vi "Actor Core.vi"(8 "error in":errorcluster, 11 "RandomDataChart in":refnum<class "ButtonPanel.lvclass">) -> (0 "error out":errorcluster, 3 "Actor out":refnum<class "Actor.lvclass">)   [LabVIEW 2015, in "TestActors.lvlib" / "ButtonPanel.lvclass"]
doc: "(<B>Filename</B>: Actor Framework.lvlib:Actor.lvclass:Actor Core.vi)\n\nReceives messages to the actor, reacts to them, and initiates any error handling that may shut the actor down.\n\nDescendant classes may override this VI to append parallel tasks for the actor to complete while it handles messages. Overrides use the Call Parent Method node."
uses:
  ButtonPanel.lvclass
  <vilib>/ActorFramework/Actor/Actor.lvclass
  <vilib>/ActorFramework/Actor/Actor.lvclass/Actor.ctl
  <vilib>/ActorFramework/Message Enqueuer/Message Enqueuer.lvclass/Message Enqueuer.ctl
  <vilib>/ActorFramework/Message Enqueuer/Init from Existing Queue.vi
  IViewable/IViewable/IViewable.lvclass
  <vilib>/ActorFramework/Message Enqueuer/Message Enqueuer.lvclass
  IViewable/IViewable Messages/Broadcast Boolean Msg/Broadcast Boolean Msg.lvclass
panel:
  in  "Launch Dialog":bool
  in  "Guthrie":bool
  in  "Harrelson":bool
  in  "Gump":bool
  in  "Wilson":bool
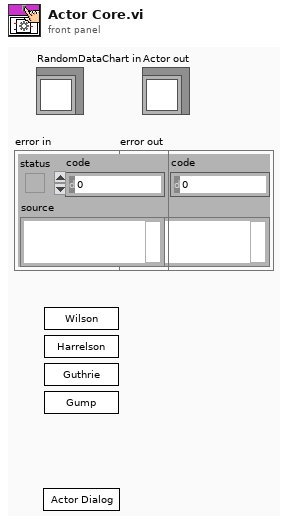
[diagram p1: front panel]
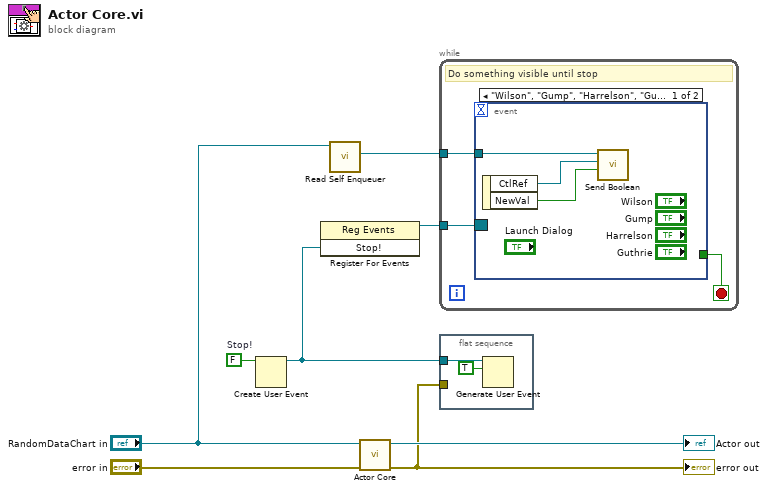
[diagram p0: block diagram]
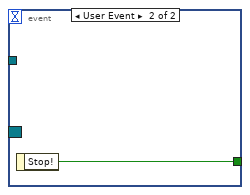
[diagram p2: hidden frame]
diagram:
  w6 = FALSE  # Stop!
  n1 = Create User Event(user event datatype=w6) -> (user event=w3:refnum<user-event>)  [unwired: 1 in, 1 out]
  n2 = register-events(w3) -> (reference out=w4:refnum<event-registration>)  [unwired: 2 in, 1 out]
  n3 = call <vilib>:"Read Self Enqueuer.vi"("Actor"="RandomDataChart in") -> ("Self Enqueuer"=w1:refnum<class "Message Enqueuer.lvclass">)  [unwired: 10 in]
  n4 = call-parent "Actor Core.vi"("error in"="error in", "IViewable In"="RandomDataChart in") -> ("error out"=w5:errorcluster, "Actor out"=→"Actor out":refnum<class "Actor.lvclass">)  [unwired: 8 in]
  "error out" <- w5
  n5 = while {
    tunnel: w4 -> [w11]
    tunnel: w1 -> [w9]
    stop <- w10 stop-if-true
    # "Do something visible until stop"
    n6 = event shown="[0] \"Wilson\", \"Gump\", \"Harrelson\", \"Guthrie\", \"Launch Dialog\": Value Change" {
      selector: w11 -> [_ _]
      dyn-events: _ -> [_ _]
      timeout: _ -> [_ _]
      tunnel: [_ w15] -> w10
      tunnel: w9 -> [w14 _]
      event "Wilson", "Gump", "Harrelson", "Guthrie", "Launch Dialog": Value Change {
        n7 = event-data() -> ("CtlRef"=w12:refnum<vi>, "NewVal"=w13:bool)  [unwired: 1 in]
        n8 = call "Send Boolean.vi"("Value"=w13, "Bool Refnum"=w12, "Message Enqueuer in"=w14) -> ()  [unwired: 8 in, 1 out]
      }
      event User Event {
        n9 = event-data() -> ("Stop!"=w15:bool)  [unwired: 1 in]
      }
    }
  }
  n10 = flat-sequence {
    tunnel: w3 -> [w17]
    tunnel: w5 -> [_]
    frame #0 {
      n11 = Generate User Event(user event=w17, event data cluster=TRUE ("event data")) -> ()  [unwired: 2 in, 2 out]
    }
  }
